vi "GetApp.vi"(0 "Project Name (\"\": ThisApplication)":string, 5 "Port(0:Ignored)":u16, 7 "Service Name (\"\":localhost)":string, 9 "Timeout ms (60000)":i32=60000, 11 "error in (no error)":errorcluster) -> (4 "Application Ref":refnum<vi>, 15 "error out":errorcluster)   [LabVIEW 2016, in "Drona.lvlib"]
doc: "Gives the reference of the application specified"
uses:
  Drona.lvlib
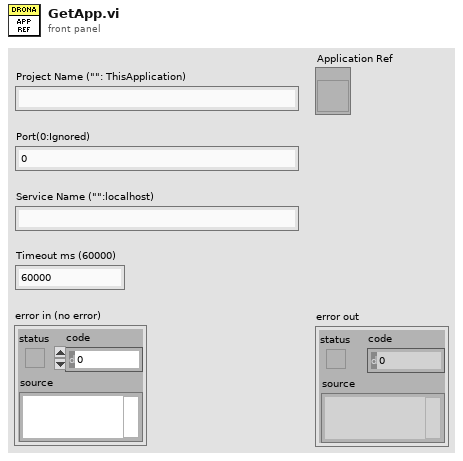
[diagram p1: front panel]
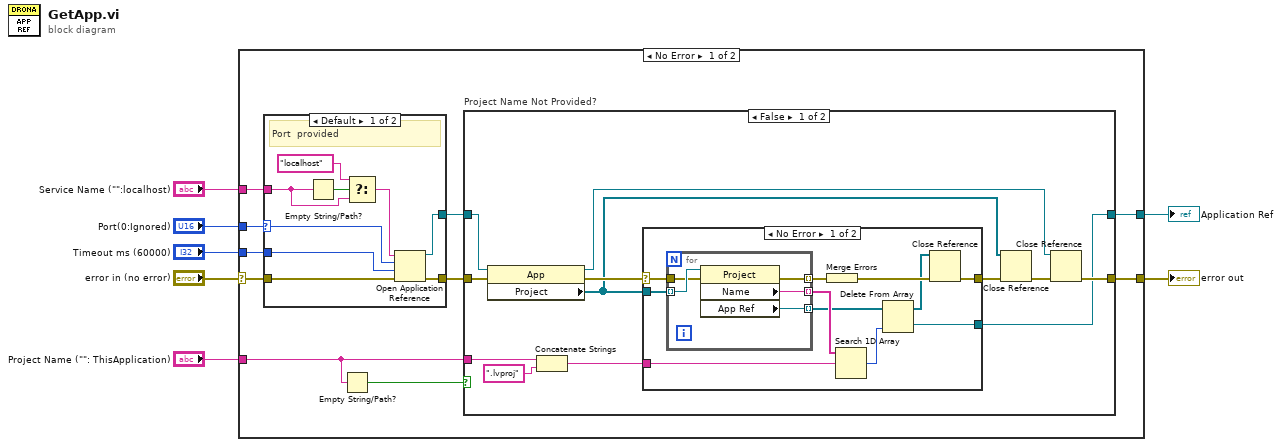
[diagram p0: block diagram]
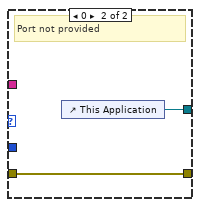
[diagram p4: hidden frame]
diagram:
  n1 = case shown="No Error" "error in (no error)" {
    selector: "error in (no error)" -> [w9 w60]
    tunnel: [w15 w60] -> w6
    tunnel: "Service Name (\"\":localhost)" -> [w13 _]
    tunnel: "Port(0:Ignored)" -> [w12 _]
    tunnel: "Project Name (\"\": ThisApplication)" -> [w11 _]
    tunnel: "Timeout ms (60000)" -> [w10 _]
    tunnel: [w8 _] -> w1
    frame No Error {
      n2 = case shown="Default" w12 {
        selector: w12 -> [w57 _]
        tunnel: w10 -> [w56 _]
        tunnel: w9 -> [w55 w59]
        tunnel: [w50 w59] -> w16
        tunnel: w13 -> [w53 _]
        tunnel: [w49 w58] -> w14
        frame Default {
          # "Port  provided"
          n3 = Empty String/Path?(string/path=w53) -> (empty?=w54:bool)
          n4 = Select(t="localhost", s=w54, f=w53) -> (s? t:f=w51:string)
          n5 = Open Application Reference(8:w55, 9:w56, 10:w57, 11:w51) -> (0:w50:errorcluster, 3:w49:refnum<vi>)
        }
        frame 0 {
          # "Port not provided"
          n6 = control-ref of="This Application"() -> (w58:refnum<vi>)
        }
      }
      n7 = Empty String/Path?(string/path=w11) -> (empty?=w17:bool)
      n8 = case "Project Name Not Provided?" shown="False" w17 {
        tunnel: w11 -> [w23 _]
        tunnel: w16 -> [w28 w48]
        tunnel: [w29 w48] -> w15
        tunnel: [w26 w47] -> w8
        tunnel: w14 -> [w25 w47]
        frame False {
          n9 = property class="App"(reference=w25, error in=w28) -> (reference out=w24:refnum<vi>, error out=w22:errorcluster, "Project"=w20:refnum<vi>[])
          n10 = Concatenate Strings(w23, ".lvproj" ("string")) -> (w19:string)
          n11 = case shown="No Error" w22 {
            selector: w22 -> [w39 w46]
            tunnel: w20 -> [w40 _]
            tunnel: [w32 w46] -> w21
            tunnel: w19 -> [w37 _]
            tunnel: [w30 _] -> w26
            frame No Error {
              n12 = for {
                tunnel: w40 -> [w45] mode=indexing
                tunnel: w39 -> [w44]
                tunnel: [w43] -> w36 mode=indexing
                tunnel: [w42] -> w38 mode=indexing
                tunnel: [w41] -> w35 mode=indexing
                n13 = property class="Project"(reference=w45, error in=w44) -> (error out=w41:errorcluster, "Name"=w42:string, "App Ref"=w43:refnum<vi>)  [unwired: 1 out]
              }
              n14 = Merge Errors(w35) -> (w34:errorcluster)
              n15 = Search 1D Array(1D array=w38, element=w37) -> (index of element=w33:i32)  [unwired: 1 in]
              n16 = Delete From Array(array=w36, index=w33) -> (deleted portion=w30:refnum<vi>, array with subset deleted=w31:refnum<vi>[])  [unwired: 1 in]
              n17 = Close Reference(reference=w31, error in (no error)=w34) -> (error out=w32:errorcluster)
            }
            frame Error {
            }
          }
          n18 = Close Reference(reference=w20, error in (no error)=w21) -> (error out=w27:errorcluster)
          n19 = Close Reference(reference=w24, error in (no error)=w27) -> (error out=w29:errorcluster)
        }
        frame True {
        }
      }
    }
    frame Error {
    }
  }
  "error out" <- w6
  "Application Ref" <- w1
